vi "compileScript.vi"(8 "error in (no error)":errorcluster, 9 "timeStamp":string, 10 "Path":path, 11 "HWController in":refnum<class "HWController.lvclass">) -> (0 "error out":errorcluster, 1 "doChannels":refnum<class "DigitalOutput.lvclass">[](array[class]), 2 "aoChannels":refnum<class "AnalogOutput.lvclass">[](array[class]), 3 "HWController out":refnum<class "HWController.lvclass">)   [LabVIEW 2009, in "Hardware.lvlib" / "HWControllers.lvlib" / "HWController.lvclass"]
uses:
  HWController.lvclass
  Channels/VoltOutput/AnalogOutput.lvclass
  Channels/Digital/DigitalOutput.lvclass
  Tools/DataMappers/DeviceData/DeviceData.lvclass
  Tools/DataMappers/DeviceData/DoDeviceData/DoDeviceData.lvclass
  Tools/DataMappers/DeviceData/AoDeviceData/AoDeviceData.lvclass
  Tools/SettingsProcessors/ScriptListCompiler/ScriptListCompiler.lvclass
  Tools/DatabaseHelpers/Database Objects/DeviceArray/DeviceArray.lvclass
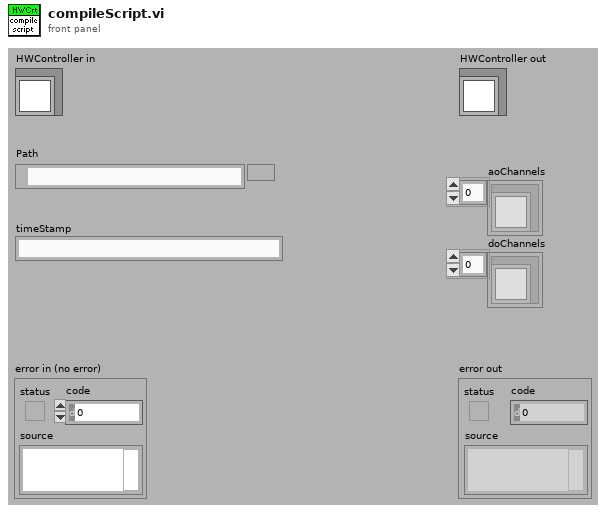
[diagram p1: front panel]
types:
  T1 = enum16{"digitalOutput", "digitalInput", "analogOutput", "analogInput", "rfOutput", "ethernetSupply"}
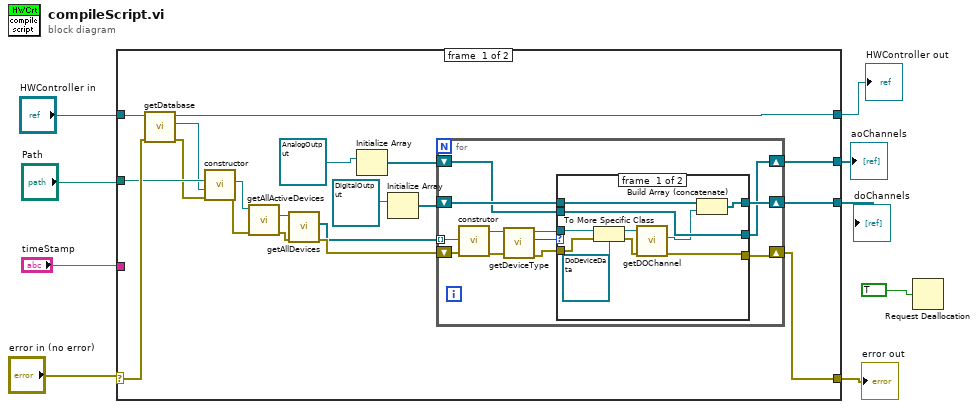
[diagram p0: block diagram]
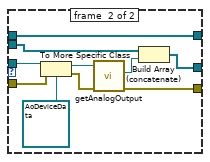
[diagram p2: hidden frame]
diagram:
  n1 = case shown="No Error" "error in (no error)" {
    selector: "error in (no error)" -> [w27 w62]
    tunnel: [w10 w62] -> w8
    tunnel: [w11 w61] -> w6
    tunnel: "HWController in" -> [w28 w61]
    tunnel: "Path" -> [w26 _]
    tunnel: "timeStamp" -> [_ _]
    tunnel: [w17 _] -> w3
    tunnel: [w16 _] -> w2
    frame #0 {
      n2 = call "getDatabase.vi"("error in (no error)"=w27, "HWController in"=w28) -> ("error out"=w24:errorcluster, "deviceDataBase"=w25:refnum<class "deviceDataBase.lvclass">, "HWController out"=w11:refnum<class "HWController.lvclass">)  [unwired: 7 in]
      n3 = call "constructor.vi"("error in (no error)"=w24, "deviceDataBase"=w25, "Path"=w26) -> ("error out"=w20:errorcluster, "DeviceArray"=w23:refnum<class "DeviceArray.lvclass">)  [unwired: 5 in, 2 out]
      n4 = call "getAllActiveDevices.vi"("error in (no error)"=w20, "DeviceArray in"=w23) -> ("error out"=w21:errorcluster, "DeviceArray"=w22:refnum<class "DeviceArray.lvclass">)  [unwired: 7 in, 1 out]
      n5 = call "getAllDevices.vi"("error in (no error)"=w21, "DeviceArray.lvclass in"=w22) -> ("error out"=w19:errorcluster, "deviceArray"=w18:refnum<class "device.lvclass">[])  [unwired: 7 in, 1 out]
      n6 = Initialize Array(refnum<class "AnalogOutput.lvclass"> refnum ("aOChannel")) -> (w14:refnum<class "AnalogOutput.lvclass">[])  [unwired: 1 in]
      n7 = Initialize Array(refnum<class "DigitalOutput.lvclass"> refnum ("DigitalOutput")) -> (w13:refnum<class "DigitalOutput.lvclass">[])  [unwired: 1 in]
      n8 = for {
        shift-right: [w30] -> w10
        shift-left: w19 -> [w40]
        shift-right: [w35] -> w16
        shift-left: w13 -> [w34]
        shift-right: [w33] -> w17
        shift-left: w14 -> [w32]
        tunnel: w18 -> [w29] mode=indexing
        n9 = call "construtor.vi"("error in (no error)"=w40, "device"=w29) -> ("error out"=w39:errorcluster, "DeviceData out"=w38:refnum<class "DeviceData.lvclass">)  [unwired: 8 in]
        n10 = call-dynamic "getDeviceType.vi"("error in (no error)"=w39, "DeviceData in"=w38) -> ("error out"=w31:errorcluster, "type"=w37:T1, "DeviceData out"=w36:refnum<class "DeviceData.lvclass">)  [unwired: 7 in]
        n11 = case shown="\"analogOutput\"" w37 {
          tunnel: w36 -> [w50 w59]
          tunnel: [w43 w56] -> w35
          tunnel: w34 -> [w42 w56]
          tunnel: [w47 w51] -> w33
          tunnel: w32 -> [w47 w53]
          tunnel: w31 -> [w46 w55]
          tunnel: [w44 w54] -> w30
          frame #0 {
            n12 = To More Specific Class(target class=refnum<class "DoDeviceData.lvclass"> refnum ("DoDeviceData.lvclass in"), reference=w50, error in=w46) -> (specific class reference=w48:refnum<class "DoDeviceData.lvclass">, error out=w45:errorcluster)
            n13 = call "getDOChannel.vi"("error in (no error)"=w45, "DoDeviceData.lvclass in"=w48) -> ("error out"=w44:errorcluster, "DigitalOutput"=w41:refnum<class "DigitalOutput.lvclass">)  [unwired: 7 in, 1 out]
            n14 = Build Array (concatenate)(w42, w41) -> (w43:refnum<class "DigitalOutput.lvclass">[])
          }
          frame #1 {
            n15 = To More Specific Class(target class=refnum<class "AoDeviceData.lvclass"> refnum ("AoDeviceData.lvclass in"), reference=w59, error in=w55) -> (specific class reference=w57:refnum<class "AoDeviceData.lvclass">, error out=w60:errorcluster)
            n16 = call "getAnalogOutput.vi"("error in (no error)"=w60, "AoDeviceData.lvclass in"=w57) -> ("error out"=w54:errorcluster, "aOChannel"=w52:refnum<class "AnalogOutput.lvclass">)  [unwired: 7 in, 1 out]
            n17 = Build Array (concatenate)(w53, w52) -> (w51:refnum<class "AnalogOutput.lvclass">[])
          }
        }
      }
    }
    frame #1 {
    }
  }
  "error out" <- w8
  "HWController out" <- w6
  "aoChannels" <- w3
  "doChannels" <- w2
  n18 = Request Deallocation(TRUE) -> ()
